vi "Var_serrure.vi"() -> ()   [LabVIEW 2018]
panel:
  in  "MAX":dbl=5.0
  out "NB_RAND":ext
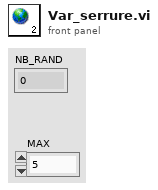
[diagram p1: front panel]
diagram:
